vi "Spectrograph_logEvent_reportedFilterPosition.vi"(8 "error in (no error)":errorcluster, 11 "logevent_reportedFilterPosition_Ctl":T1) -> (0 "error out":errorcluster, 2 "function return":i32, 3 "logevent_reportedFilterPosition_Ctl out":T1)   [LabVIEW 2016, in "SALLV_Spectrograph.lvlib"]
doc: "int Spectrograph_shm_logEvent_reportedFilterPositionLV(Spectrograph_logevent_reportedFilterPositionLV *logevent_reportedFilterPosition_Ctl );"
uses:
  SALLV_Spectrograph.lvlib
  DataTypes/logevent_reportedFilterPosition.ctl
  SALLV_Spectrograph.so
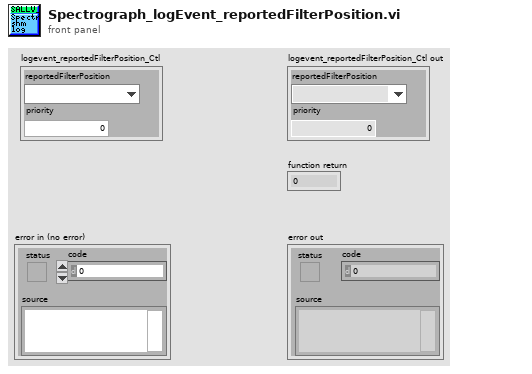
[diagram p1: front panel]
types:
  T1 = typedef "SALLV_Spectrograph.lvlib/logevent_reportedFilterPosition.ctl" = cluster{"reportedFilterPosition":enum32{"", "filter0", "filter1", "filter2", "filter3", "filter4"}, "priority":i32}
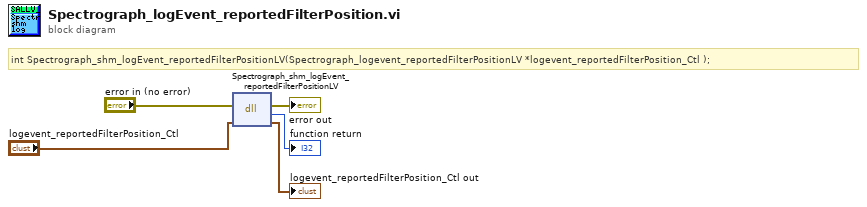
[diagram p0: block diagram]
diagram:
  # "int Spectrograph_shm_logEvent_reportedFilterPositionLV(Spectrograph_logevent_reportedFilterPositionLV *logevent_reportedFilterPosition_Ctl );"
  n1 = dll-call lib="home/harini/TCS/SALLV_Spectrograph/SALLV_Spectrograph.*" fn="Spectrograph_shm_logEvent_reportedFilterPositionLV"(error in="error in (no error)", "logevent_reportedFilterPosition_Ctl"="logevent_reportedFilterPosition_Ctl") -> (error out=→"error out":errorcluster, →"function return":i32, "logevent_reportedFilterPosition_Ctl"=→"logevent_reportedFilterPosition_Ctl out":T1)  [unwired: 2 in, 1 out]
